vi "App.Initialize.vi"(8 "error in (no error)":errorcluster, 11 "Start Variables":T1) -> (0 "error out":errorcluster)   [LabVIEW 2013, in "Simple Sequence Editor.lvlib"]
uses:
  Simple Sequence Editor.lvlib
  Types/StateVariables.ctl
  Types/ChannelProperties.ctl
  Types/UI.PropertiesTypes.ctl
  Constants.vi
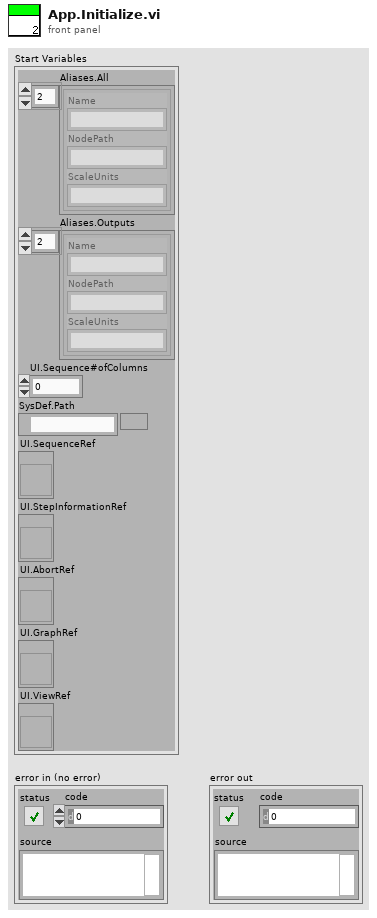
[diagram p1: front panel]
types:
  T1 = typedef "Simple Sequence Editor.lvlib/StateVariables.ctl" = cluster{"Aliases.All":T2[], "Aliases.Outputs":T2[], "UI.Sequence#ofColumns":i32, "SysDef.Path":path, "UI.SequenceRef":refnum<vi>, "UI.StepInformationRef":refnum<vi>, "UI.AbortRef":refnum<vi>, "UI.GraphRef":refnum<vi>, "UI.ViewRef":refnum<vi>}
  T2 = typedef "Simple Sequence Editor.lvlib/ChannelProperties.ctl" = cluster{"Name":string, "NodePath":string, "ScaleUnits":string}
  T3 = typedef "Simple Sequence Editor.lvlib/UI.PropertiesTypes.ctl" = enum8{"Step Properties", "Sequence Properties"}
  T4 = typedef "LVBoundsTypeDef.ctl" = cluster{"Width":u32, "Height":u32}
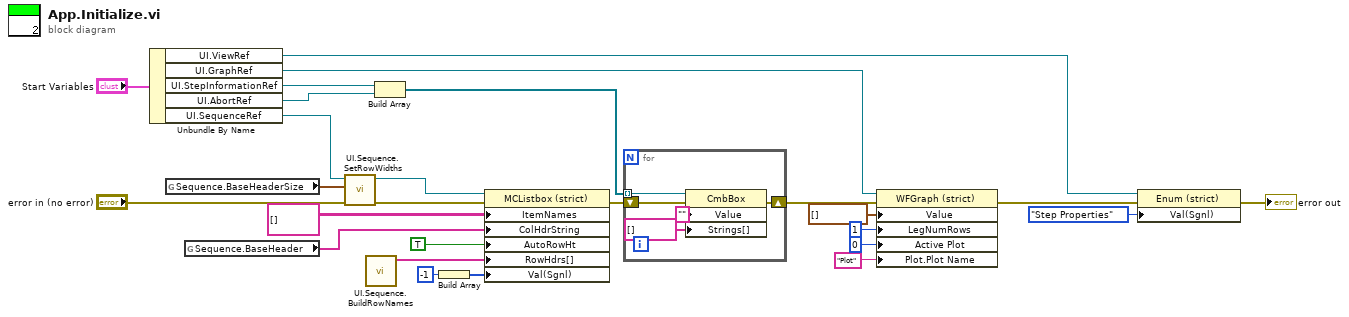
[diagram p0: block diagram]
diagram:
  n1 = Unbundle By Name("Start Variables") -> ("UI.ViewRef"=w22:refnum<vi>, "UI.GraphRef"=w16:refnum<vi>, "UI.StepInformationRef"=w14:refnum<vi>, "UI.AbortRef"=w13:refnum<vi>, "UI.SequenceRef"=w8:refnum<vi>)
  n2 = global read "Constants.vi" "Sequence.BaseHeaderSize"() -> (w1:T4[])
  n3 = global read "Constants.vi" "Sequence.BaseHeader"() -> (w2:string[])
  n4 = call "UI.Sequence.SetRowWidths.vi"("error in (no error)"="error in (no error)", "Array"=w1, "UI.SequenceRef"=w8) -> ("error out"=w7:errorcluster, "UI.SequenceRef"=w9:refnum<vi>)  [unwired: 7 in]
  n5 = call "UI.Sequence.BuildRowNames.vi"() -> ("Array"=w10:string[])  [unwired: 11 in]
  n6 = Build Array(w14, w13) -> (w15:refnum<vi>[])
  n7 = Build Array(-1 ("Value")) -> (w12:i32[])
  n8 = property class="MCListbox (strict)"(reference=w9, error in=w7, "ItemNames"=string[][] [] ("Item Names"), "ColHdrString"=w2, "AutoRowHt"=TRUE ("Autosizing Row Height"), "RowHdrs[]"=w10, "Val(Sgnl)"=w12) -> (error out=w26:errorcluster)  [unwired: 1 out]
  n9 = for {
    tunnel: w15 -> [w30] mode=indexing
    shift-right: [w28] -> w17
    shift-left: w26 -> [w31]
    n10 = property class="CmbBox"(reference=w30, error in=w31, "Value"="", "Strings[]"=string[] [] ("Strings []")) -> (error out=w28:errorcluster)  [unwired: 1 out]
  }
  n11 = property class="WFGraph (strict)"(reference=w16, error in=w17, "Value"=waveform(dbl)[] [], "LegNumRows"=u32 1 ("Legend:Number of Rows"), "Active Plot"=u32 0, "Plot.Plot Name"="Plot") -> (error out=w23:errorcluster)  [unwired: 1 out]
  n12 = property class="Enum (strict)"(reference=w22, error in=w23, "Val(Sgnl)"=UI.PropertiesTypes."Step Properties" ("Value (Signaling)")) -> (error out=→"error out":errorcluster)  [unwired: 1 out]
